vi "Test 4 Serial Read Data is Written to Decorated Interface.vi"(8 "error in (no error)":errorcluster, 11 "Serial Logging Decorator Test In":refnum<class "Serial Logging Decorator Test.lvclass">) -> (0 "error out":errorcluster, 3 "Serial Logging Decorator Test Out":refnum<class "Serial Logging Decorator Test.lvclass">)   [LabVIEW 2020, in "Serial Logging Decorator Test.lvclass"]
uses:
  Log/Log.lvclass
  Serial Logging Decorator Test.lvclass
  Serial Logging Decorator Test.lvclass/Serial Logging Decorator Test.ctl
  Serial Logging Decorator/Serial Logging Decorator.lvclass
  Mock Serial/Mock Serial.lvclass
  Serial/Serial.lvclass/Serial.lvclass
  c550bb1f-22ef-4c0e-b612-66d7cf5e5730.vi
  C:/Program Files (x86)/National Instruments/LabVIEW 2020/vi.lib/Astemes/LMock/Mock.lvclass
  C:/git/astemes-lmock/sandbox/Examples/Mock Serial/Mock Serial.lvclass
  C:/git/astemes-lmock/sandbox/Examples/Serial/Serial.lvclass/Serial.lvclass
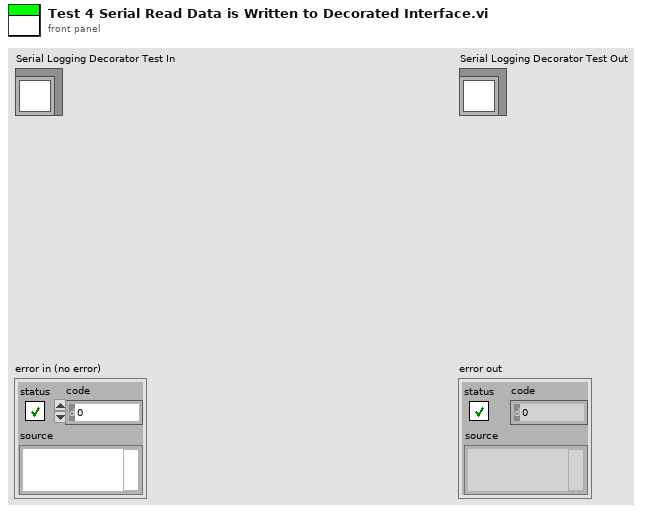
[diagram p1: front panel]
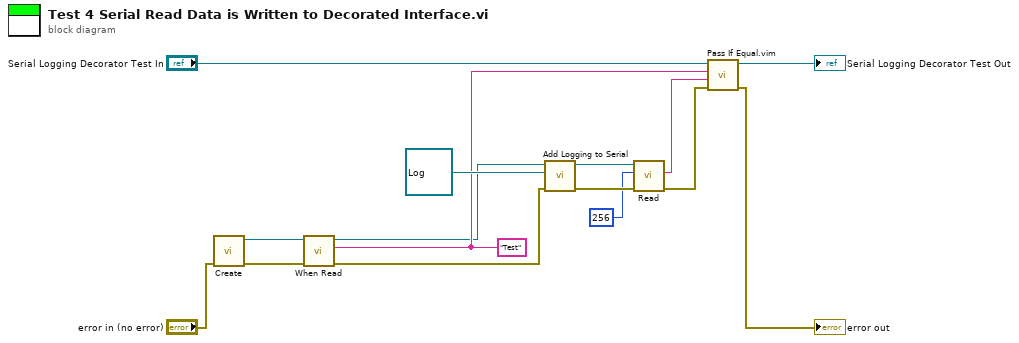
[diagram p0: block diagram]
diagram:
  w4 = "Test" ("Text to Write")
  n1 = call "Create.vi"("error in (no error)"="error in (no error)") -> ("error out"=w1:errorcluster, "Mock Class Generator out"=w11:refnum<class "Mock Serial.lvclass">)  [unwired: 9 in]
  n2 = call "When Read.vi"("error out"=w1, "read buffer"=w4, "Serial in"=w11) -> ("Serial out"=w3:refnum<class "Mock Serial.lvclass">)  [unwired: 8 in]
  n3 = call "Add Logging to Serial.vi"("error in (no error)"=w1, "Log Destination"=refnum<class "Log.lvclass"> refnum ("Log.lvclass"), "Serial"=w3) -> ("error out"=w9:errorcluster, "Serial with Logging"=w10:refnum<class "Serial.lvclass">)  [unwired: 7 in]
  n4 = call-dynamic "Read.vi"("error in (no error)"=w9, "byte count"=u32 256, "Serial in"=w10) -> ("error out"=w7:errorcluster, "read buffer"=w5:string)  [unwired: 6 in, 1 out]
  n5 = call "Pass If Equal.vim"("error in (no error)"=w7, "Actual"=w5, "Expected"=w4, "LUnit Test Case In"="Serial Logging Decorator Test In") -> ("error out"=→"error out":errorcluster, "LUnit Test Case Out"=→"Serial Logging Decorator Test Out":refnum<class "Serial Logging Decorator Test.lvclass">)  [unwired: 6 in]
